vi "one_channel_send_read.vi"() -> ()   [LabVIEW 2022 SP3]
uses:
  <instrlib>/Tektronix DPO MSO 2000 4000 Series/Public/Configure/Configure Trigger (Edge).vi
  <instrlib>/Tektronix AFG 3000 Series/Tektronix AFG 3000 Series.lvlib
  <instrlib>/Tektronix DPO MSO 2000 4000 Series/Tektronix DPO MSO 2000 4000 Series.lvlib
panel:
  in  "Enable Output":bool=TRUE
  in  "DC Offset (0.00 V)":dbl
  in  "Amplitude (1 Vpp)":dbl=1.0
  in  "Waveform Function (0: Sine)":u16(ring) items=["Sine", "Square", "Pulse", "Ramp", "Noise", "DC", "Sin(x)/x", "Gaussian", "Lorentz", "Exponential Rise", "Exponential Decay", "Haversine"]
  in  "Frequency (1000 Hz)":dbl=1000.0
  in  "Record Length (10: 10k points)":u32(ring)=10 items=["1000 points"=1, "10k points"=10, "100k points"=100, "1M points"=1000, "10M points"=10000]
  in  "Maximum Time (10000ms)":u32=10000
  in  "Vertical Coupling (1: DC)":u16(ring)=1 items=["AC", "DC", "Ground"]
  in  "Oscope Name":refnum<visa-resource-name>
  in  "Oscope Wave Channel":u16(ring) items=["Channel 1", "Channel 2", "Channel 3", "Channel 4", "Math", "Reference 1", "Reference 2", "Reference 3", "Reference 4"]
  in  "Trigger Level (0.0)":dbl
  in  "Timebase (4.0e-5)":dbl=4e-05
  in  "Vertical Range (1.0)":dbl=1.0
  in  "Vertical Offset (0)":dbl
  out "Waveform Graph":waveform(dbl)(graph)
  in  "Burst Mode (0: Triggered)":u16(ring) items=["Triggered", "Gated"]
  in  "FN Wave Channel":u16(ring) items=["Channel 1", "Channel 2"]
  in  "Internal Trigger Rate (500)":dbl=500.0
  in  "Burst Count (5)":i32=5
  in  "FN Generator Name":refnum<visa-resource-name>
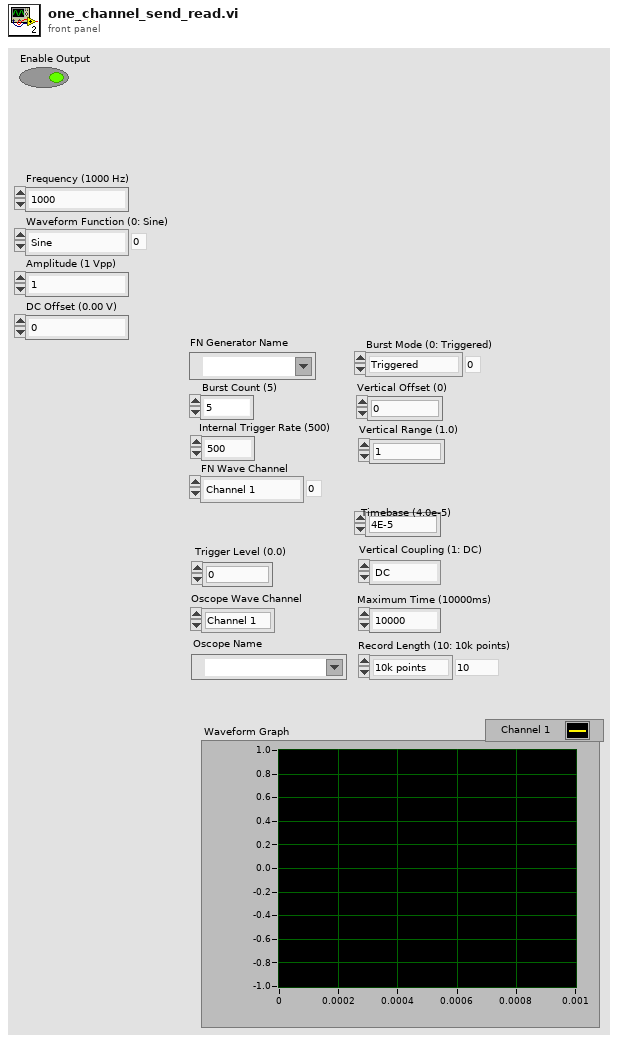
[diagram p1: front panel]
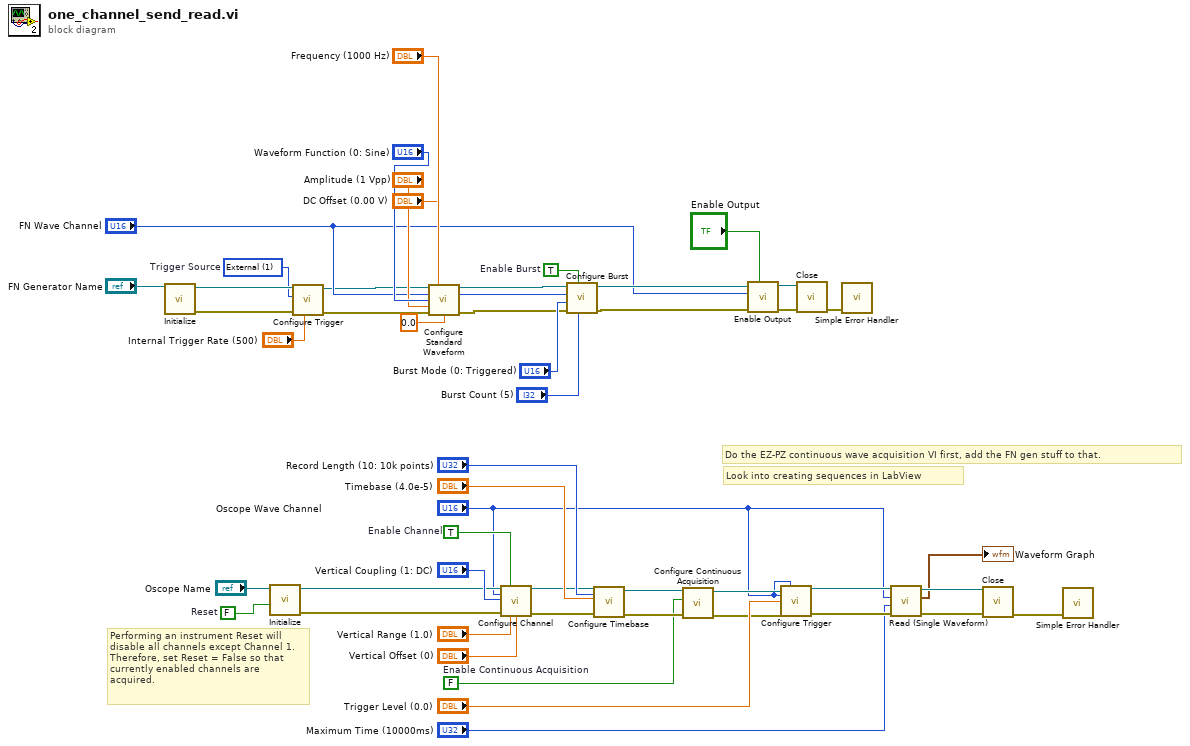
[diagram p0: block diagram]
diagram:
  w20 = FALSE  # Enable Continuous Acquisition
  w15 = TRUE  # Enable Channel
  w25 = FALSE  # Reset
  w39 = u16 1 items=["Internal"=3, "External"=1]  # Trigger Source
  w43 = TRUE  # Enable Burst
  # "Look into creating sequences in LabView"
  # "Do the EZ-PZ continuous wave acquisition VI first, add the FN gen stuff to that."
  # "Performing an instrument Reset will disable all channels except Channel 1. Therefore, set Reset = False so that currently enabled channels are acquired."
  n1 = call <instrlib>:"Initialize.vi"("VISA resource name"="FN Generator Name") -> ("error out"=w40:errorcluster, "VISA resource name out"=w41:refnum<visa-resource-name>)  [unwired: 9 in]
  n2 = call <instrlib>:"Initialize.vi"("Reset (True)"=w25, "VISA resource name"="Oscope Name") -> ("error out"=w16:errorcluster, "VISA resource name out"=w17:refnum<visa-resource-name>)  [unwired: 8 in]
  n3 = call <instrlib>:"Configure Trigger.vi"("Internal Trigger Rate (500)"="Internal Trigger Rate (500)", "error in (no error)"=w40, "Trigger Source (3:Internal)"=w39, "VISA resource name"=w41) -> ("error out"=w3:errorcluster, "VISA resource name out"=w7:refnum<visa-resource-name>)  [unwired: 6 in]
  n4 = call <instrlib>:"Configure Standard Waveform.vi"("VISA resource name"=w7, "Frequency (1000 Hz)"="Frequency (1000 Hz)", "Channel (0: Channel 1)"="FN Wave Channel", "Waveform Function (0: Sine)"="Waveform Function (0: Sine)", "Amplitude (1 Vpp)"="Amplitude (1 Vpp)", "error in (no error)"=w3, "DC Offset (0.00 V)"="DC Offset (0.00 V)", "Phase Level (-1)"=0.0) -> ("VISA resource name out"=w6:refnum<visa-resource-name>, "error out"=w2:errorcluster)  [unwired: 6 in]
  n5 = call <instrlib>:"Configure Channel.vi"("VISA resource name"=w17, "Enable Channel (T: Enable)"=w15, "Channel (0: Channel 1)"="Oscope Wave Channel", "Vertical Coupling (1: DC)"="Vertical Coupling (1: DC)", "error in (no error)"=w16, "Vertical Range (10.0 V)"="Vertical Range (1.0)", "Vertical Offset (0.0 V)"="Vertical Offset (0)") -> ("VISA resource name out"=w24:refnum<visa-resource-name>, "error out"=w23:errorcluster)  [unwired: 7 in]
  n6 = call <instrlib>:"Configure Burst.vi"("Burst Count (5)"="Burst Count (5)", "Enable Burst (T: Enable)"=w43, "error in (no error)"=w2, "Burst Mode (0: Triggered)"="Burst Mode (0: Triggered)", "Channel (0: Channel 1)"="FN Wave Channel", "VISA resource name"=w6) -> ("error out"=w49:errorcluster, "VISA resource name out"=w50:refnum<visa-resource-name>)  [unwired: 4 in]
  n7 = call <instrlib>:"Configure Timebase.vi"("Record Length (10: 10k points)"="Record Length (10: 10k points)", "error in (no error)"=w23, "Timebase (0.0005 s)"="Timebase (4.0e-5)", "VISA resource name"=w24) -> ("error out"=w21:errorcluster, "VISA resource name out"=w22:refnum<visa-resource-name>)  [unwired: 6 in]
  n8 = call <instrlib>:"Configure Continuous Acquisition.vi"("error in (no error)"=w21, "Enable Continuous Acquisition Mode (T: Enable)"=w20, "VISA resource name"=w22) -> ("error out"=w18:errorcluster, "VISA resource name out"=w19:refnum<visa-resource-name>)  [unwired: 7 in]
  n9 = call <instrlib>:"Enable Output.vi"("Enable Output (T: Enable)"="Enable Output", "error in (no error)"=w49, "Channel (0: Channel 1)"="FN Wave Channel", "VISA resource name"=w50) -> ("error out"=w47:errorcluster, "VISA resource name out"=w48:refnum<visa-resource-name>)  [unwired: 6 in]
  n10 = call-poly <instrlib>:"Configure Trigger.vi"("VISA resource name"=w19, "Trigger Coupling (0 : DC)"="Oscope Wave Channel", "Trigger Source (0: Channel 1)"="Oscope Wave Channel", "Trigger Level (0.0 V)"="Trigger Level (0.0)", "error in (no error)"=w18) -> ("VISA resource name out"=w34:refnum<visa-resource-name>, "error out"=w29:errorcluster)  [unwired: 9 in]
  n11 = call <instrlib>:"Close.vi"("error in (no error)"=w47, "VISA resource name"=w48) -> ("error out"=w46:errorcluster)  [unwired: 9 in]
  n12 = call <vilib>:"Simple Error Handler.vi"("error in (no error)"=w46) -> ()  [unwired: 4 in, 5 out]
  n13 = call <instrlib>:"Read (Single Waveform).vi"("error in (no error)"=w29, "Maximum Time (10000ms)"="Maximum Time (10000ms)", "Channel (0: Channel 1)"="Oscope Wave Channel", "VISA resource name"=w34) -> ("error out"=w28:errorcluster, "Waveform Graph"=→"Waveform Graph":waveform(dbl), "VISA resource name out"=w32:refnum<visa-resource-name>)  [unwired: 5 in]
  n14 = call <instrlib>:"Close.vi"("error in (no error)"=w28, "VISA resource name"=w32) -> ("error out"=w33:errorcluster)  [unwired: 9 in]
  n15 = call <vilib>:"Simple Error Handler.vi"("error in (no error)"=w33) -> ()  [unwired: 4 in, 5 out]
